vi "Build Source Waveform.vi"(0 "RFFE Command in":refnum<class "RFFE Command.lvclass">, 11 "error in (no error)":errorcluster) -> (4 "RFFE Command out":refnum<class "RFFE Command.lvclass">, 6 "Source Waveform":u32[](array[numeric]), 15 "error out":errorcluster)   [LabVIEW 2018, in "MIPI RFFE API.lvlib" / "RFFE Command.lvclass"]
uses:
  RFFE Command.lvclass
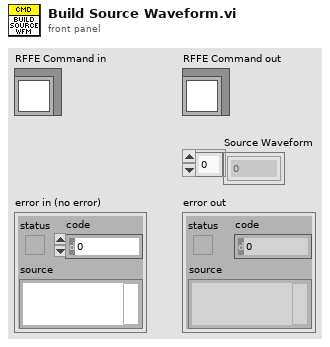
[diagram p1: front panel]
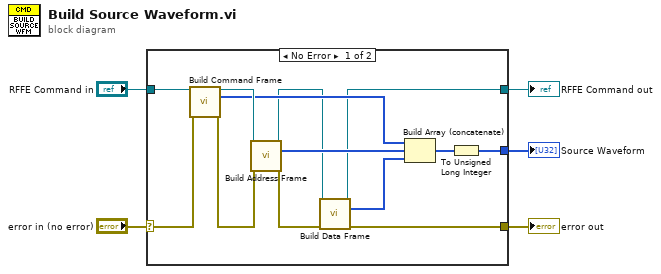
[diagram p0: block diagram]
diagram:
  n1 = case shown="No Error" "error in (no error)" {
    selector: "error in (no error)" -> [w15 w20]
    tunnel: [w7 w20] -> w4
    tunnel: [w8 w19] -> w2
    tunnel: "RFFE Command in" -> [w16 w19]
    tunnel: [w11 _] -> w1
    frame No Error {
      n2 = call-dynamic "Build Command Frame.vi"("RFFE Command in"=w16, "error in (no error)"=w15) -> ("RFFE Command out"=w18:refnum<class "RFFE Command.lvclass">, "Command Frame"=w14:u8[], "error out"=w17:errorcluster)  [unwired: 11 in]
      n3 = call-dynamic "Build Address Frame.vi"("RFFE Command in"=w18, "error in (no error)"=w17) -> ("RFFE Command out"=w10:refnum<class "RFFE Command.lvclass">, "Address Frame"=w13:u8[], "error out"=w9:errorcluster)  [unwired: 11 in]
      n4 = call-dynamic "Build Data Frame.vi"("RFFE Command in"=w10, "error in (no error)"=w9) -> ("RFFE Command out"=w8:refnum<class "RFFE Command.lvclass">, "Data Frame"=w6:u8[], "error out"=w7:errorcluster)  [unwired: 11 in]
      n5 = Build Array (concatenate)(w14, w13, w6) -> (w12:u8[])
      n6 = To Unsigned Long Integer(number=w12) -> (unsigned 32bit integer=w11:u32[])
    }
    frame Error {
    }
  }
  "error out" <- w4
  "RFFE Command out" <- w2
  "Source Waveform" <- w1
